vi "Launch.vi"(0 "File":string, 1 "Cmd":string, 2 "Mode":u16(ring) items=["Normal", "Keep", "Hide"], 3 "Path":path) -> ()   [LabVIEW 2014]
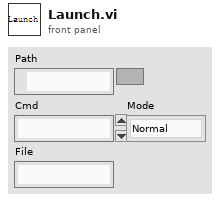
[diagram p1: front panel]
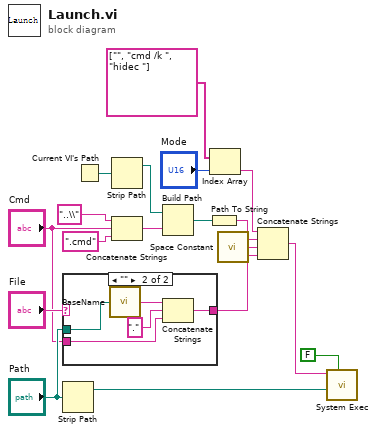
[diagram p0: block diagram]
diagram:
  n1 = case shown="\"\"" "File" {
    selector: "File" -> [w19 _]
    tunnel: "Path" -> [_ w24]
    tunnel: "Cmd" -> [_ w23]
    tunnel: [w19 w22] -> w7
    frame Default {
    }
    frame "" {
      n2 = call "BaseName.vi"("Path"=w24) -> ("Name"=w21:string)
      n3 = Concatenate Strings(w21, "." ("string"), w23) -> (w22:string)
    }
  }
  n4 = Strip Path(path="Path") -> (stripped path=w15:path)  [unwired: 1 out]
  n5 = Current VI's Path() -> (path=w17:path)
  n6 = Strip Path(path=w17) -> (stripped path=w16:path)  [unwired: 1 out]
  n7 = Concatenate Strings("..\\" ("name or relative path"), "Cmd", ".cmd" ("string")) -> (w9:string)
  n8 = Build Path(base path=w16, name or relative path=w9) -> (appended path=w14:path)
  n9 = Path To String(path=w14) -> (string=w5:string)
  n10 = Index Array(array=string[] ["", "cmd /k ", "hidec "], index="Mode") -> (element=w1:string)
  n11 = call <vilib>:"Space Constant.vi"() -> ("String"=w6:string)
  n12 = Concatenate Strings(w1, w5, w6, w7) -> (w4:string)
  n13 = call <vilib>:"System Exec.vi"("wait until completion? (T)"=FALSE, "working directory"=w15, "command line"=w4) -> ()  [unwired: 5 in, 4 out]
